vi "SistematicaAssaig.vi"(4 "Iniciar/Finalitzar":refnum<vi>, 5 "PantallaColocada":refnum<vi>, 6 "T0":refnum<vi>, 7 "Value":enum32{"Calibración", "Ensayo A", "Ensayo B"}(ring), 8 "Primera":refnum<vi>, 9 "Temperatura1":refnum<vi>, 10 "Poner Pantalla":refnum<vi>, 11 "DisparoPantalla":refnum<vi>) -> ()   [LabVIEW 2017]
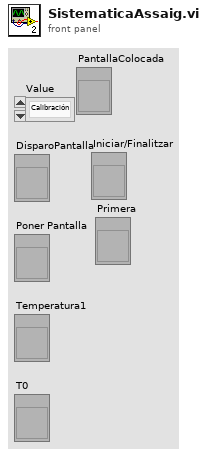
[diagram p1: front panel]
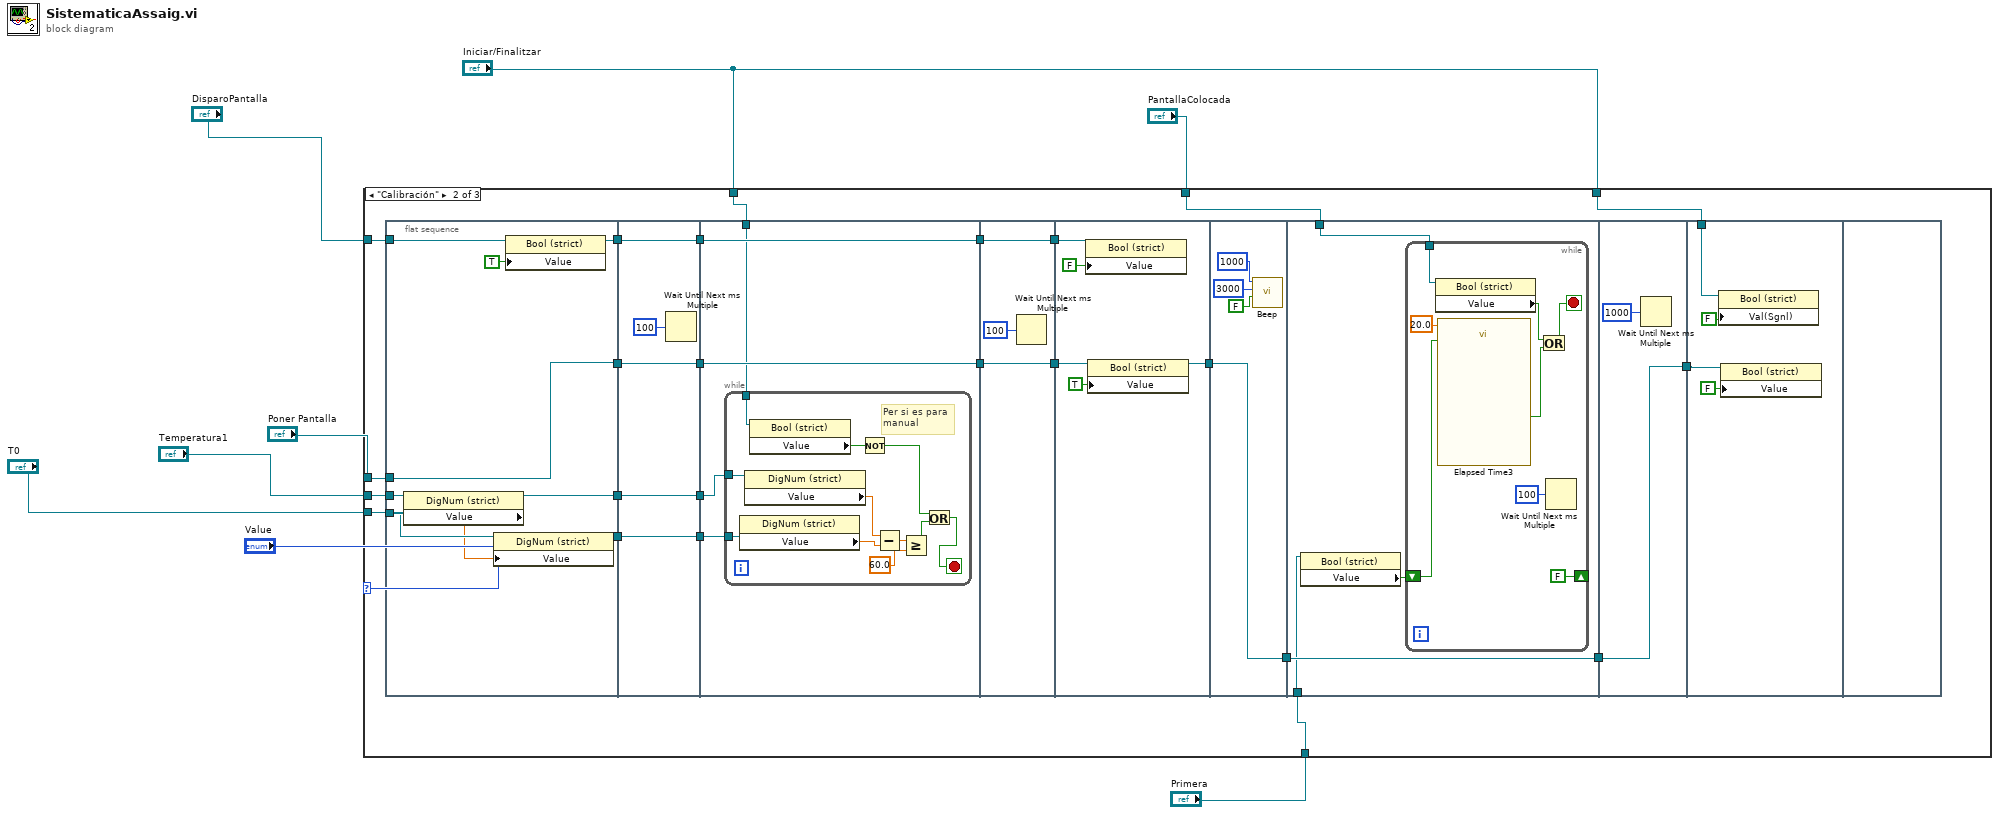
[diagram p0: block diagram]
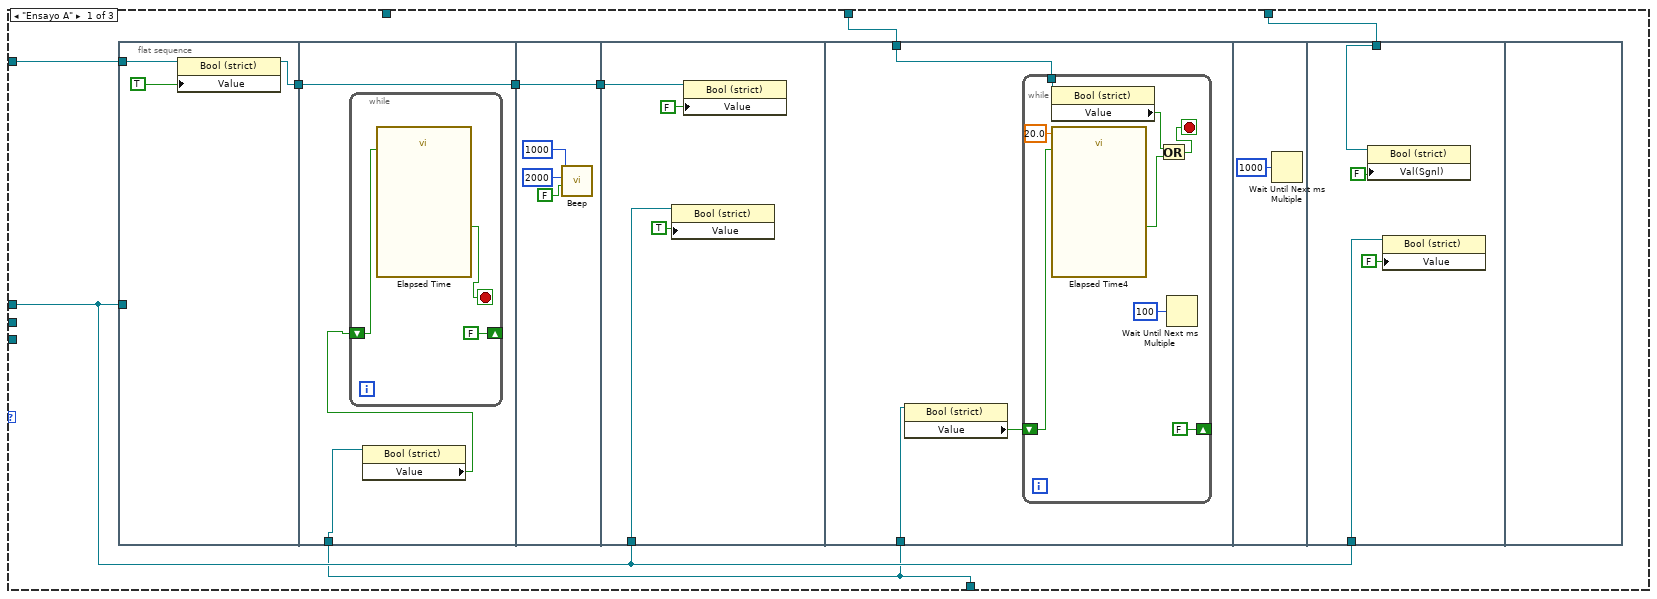
[diagram p2: hidden frame]
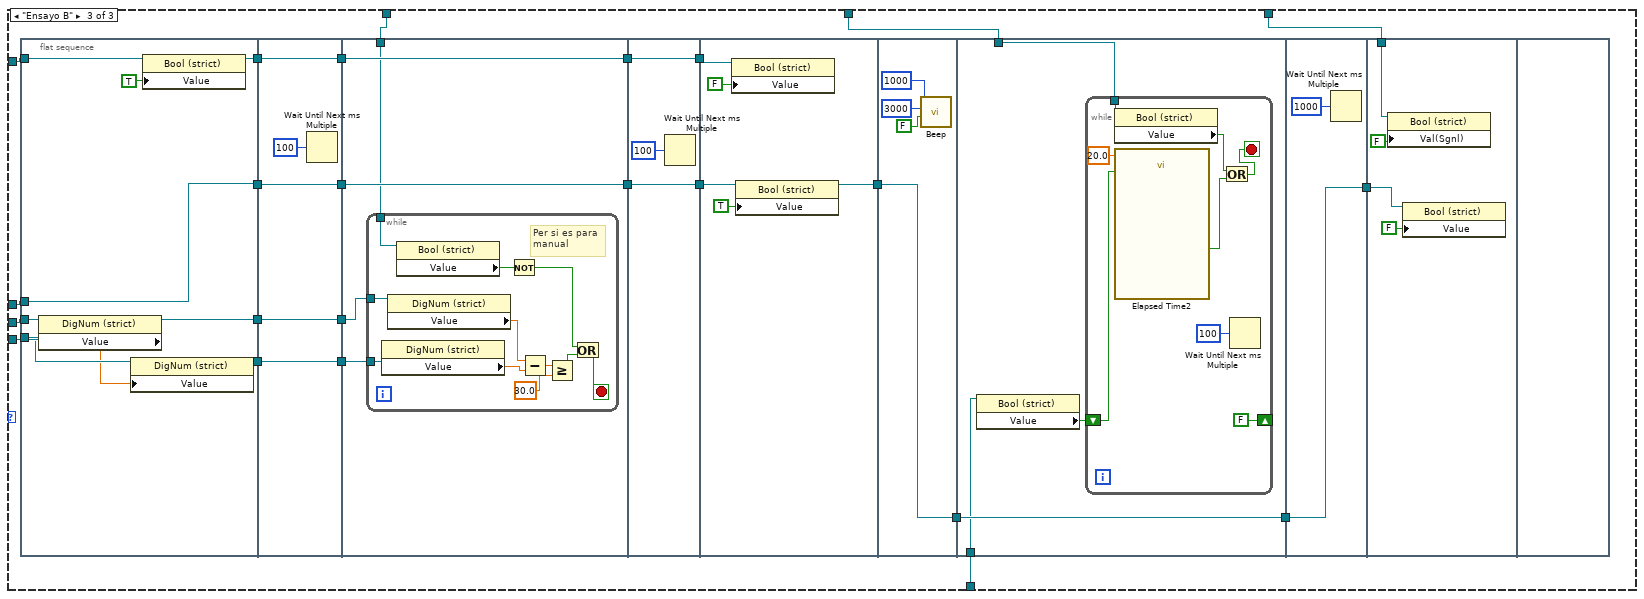
[diagram p3: hidden frame]
diagram:
  n1 = case shown="\"Calibración\"" "Value" {
    tunnel: "DisparoPantalla" -> [w16 w73 w157]
    tunnel: "Poner Pantalla" -> [w10 w71 w155]
    tunnel: "Temperatura1" -> [_ w72 w156]
    tunnel: "T0" -> [_ w70 w154]
    tunnel: "Iniciar/Finalitzar" -> [w11 w68 w152]
    tunnel: "PantallaColocada" -> [w12 w69 w153]
    tunnel: "Iniciar/Finalitzar" -> [_ w53 w137]
    tunnel: "Primera" -> [w9 w50 w134]
    frame "Ensayo A" {
      n2 = flat-sequence {
        tunnel: w16 -> [w19]
        tunnel: [w17] -> w13
        tunnel: w10 -> [_]
        tunnel: [w22] -> w14
        tunnel: w13 -> [w22]
        tunnel: w9 -> [w21]
        tunnel: [w26] -> w15
        tunnel: w14 -> [w26]
        tunnel: w15 -> [w33]
        tunnel: w10 -> [w31]
        tunnel: w12 -> [w36]
        tunnel: w9 -> [w35]
        tunnel: w11 -> [w47]
        tunnel: w10 -> [w46]
        frame #0 {
          n3 = property class="Bool (strict)"(reference=w19, "Value"=TRUE ("Reset_Time")) -> (reference out=w17:refnum<vi>)  [unwired: 1 in, 1 out]
        }
        frame #1 {
          n4 = property class="Bool (strict)"(reference=w21) -> ("Value"=w20:bool)  [unwired: 1 in, 2 out]
          n5 = while {
            shift-right: [FALSE ("Value")] -> _
            shift-left: w20 -> [w23]
            stop <- w25 stop-if-true
            n6 = call "Elapsed Time"("Reset"=w23) -> ("Time has Elapsed"=w25:bool)  [unwired: 11 in, 7 out]
          }
        }
        frame #2 {
          n7 = call <vilib>:"Beep.vi"("use system alert? (T)"=FALSE, "duration (msec)"=u32 2000, "frequency (Hz)"=u32 1000) -> ()  [unwired: 9 in]
        }
        frame #3 {
          n8 = property class="Bool (strict)"(reference=w31, "Value"=TRUE) -> ()  [unwired: 1 in, 2 out]
          n9 = property class="Bool (strict)"(reference=w33, "Value"=FALSE) -> ()  [unwired: 1 in, 2 out]
        }
        frame #4 {
          n10 = property class="Bool (strict)"(reference=w35) -> ("Value"=w34:bool)  [unwired: 1 in, 2 out]
          n11 = while {
            tunnel: w36 -> [w44]
            shift-right: [FALSE ("Value")] -> _
            shift-left: w34 -> [w37]
            stop <- w41 stop-if-true
            n12 = property class="Bool (strict)"(reference=w44) -> ("Value"=w43:bool)  [unwired: 1 in, 2 out]
            n13 = call "Elapsed Time4"("Time Target (s)"=20.0, "Reset"=w37) -> ("Time has Elapsed"=w42:bool)  [unwired: 10 in, 7 out]
            n14 = Or(x=w43, y=w42) -> (x .or. y?=w41:bool)
            n15 = Wait Until Next ms Multiple(millisecond multiple=u32 100) -> ()  [unwired: 1 out]
          }
        }
        frame #5 {
          n16 = Wait Until Next ms Multiple(millisecond multiple=u32 1000) -> ()  [unwired: 1 out]
        }
        frame #6 {
          n17 = property class="Bool (strict)"(reference=w47, "Val(Sgnl)"=FALSE ("Value (Signaling)")) -> ()  [unwired: 1 in, 2 out]
          n18 = property class="Bool (strict)"(reference=w46, "Value"=FALSE) -> ()  [unwired: 1 in, 2 out]
        }
        frame #7 {
        }
      }
    }
    frame "Calibración" {
      n19 = flat-sequence {
        tunnel: w73 -> [w82]
        tunnel: w72 -> [w81]
        tunnel: [w80] -> w67
        tunnel: w71 -> [w79]
        tunnel: [w79] -> w65
        tunnel: [w77] -> w63
        tunnel: w70 -> [w76]
        tunnel: [w74] -> w61
        tunnel: w67 -> [w87]
        tunnel: [w87] -> w66
        tunnel: w65 -> [w86]
        tunnel: [w86] -> w64
        tunnel: w63 -> [w85]
        tunnel: [w85] -> w62
        tunnel: w61 -> [w84]
        tunnel: [w84] -> w60
        tunnel: w66 -> [w92]
        tunnel: w64 -> [w91]
        tunnel: [w91] -> w59
        tunnel: w62 -> [w89]
        tunnel: w60 -> [w90]
        tunnel: [w89] -> w57
        tunnel: w53 -> [w88]
        tunnel: w59 -> [w106]
        tunnel: [w106] -> w58
        tunnel: w57 -> [w105]
        tunnel: [w105] -> w56
        tunnel: [w111] -> w52
        tunnel: w58 -> [w110]
        tunnel: w56 -> [w108]
        tunnel: w52 -> [w115]
        tunnel: [w115] -> w51
        tunnel: w69 -> [w119]
        tunnel: w51 -> [w118]
        tunnel: [w118] -> w55
        tunnel: w50 -> [w116]
        tunnel: w55 -> [w129]
        tunnel: [w129] -> w54
        tunnel: w54 -> [w132]
        tunnel: w68 -> [w131]
        frame #0 {
          n20 = property class="DigNum (strict)"(reference=w81) -> (reference out=w80:refnum<vi>, "Value"=w75:sgl)  [unwired: 1 in, 1 out]
          n21 = property class="DigNum (strict)"(reference=w76, "Value"=w75) -> (reference out=w74:refnum<vi>)  [unwired: 1 in, 1 out]
          n22 = property class="Bool (strict)"(reference=w82, "Value"=TRUE ("Reset_Time")) -> (reference out=w77:refnum<vi>)  [unwired: 1 in, 1 out]
        }
        frame #1 {
          n23 = Wait Until Next ms Multiple(millisecond multiple=u32 100) -> ()  [unwired: 1 out]
        }
        frame #2 {
          n24 = while {
            tunnel: w92 -> [w103]
            tunnel: w90 -> [w99]
            tunnel: w88 -> [w96]
            stop <- w93 stop-if-true
            # "Per si es para \nmanual"
            n25 = property class="DigNum (strict)"(reference=w99) -> ("Value"=w98:sgl)  [unwired: 1 in, 2 out]
            n26 = property class="DigNum (strict)"(reference=w103) -> ("Value"=w102:sgl)  [unwired: 1 in, 2 out]
            n27 = property class="Bool (strict)"(reference=w96) -> ("Value"=w97:bool)  [unwired: 1 in, 2 out]
            n28 = Not(x=w97) -> (.not. x?=w95:bool)
            n29 = Subtract(x=w102, y=w98) -> (x-y=w101:sgl)
            n30 = Greater Or Equal?(x=w101, y=sgl 60.0) -> (x >= y?=w94:bool)
            n31 = Or(x=w95, y=w94) -> (x .or. y?=w93:bool)
          }
        }
        frame #3 {
          n32 = Wait Until Next ms Multiple(millisecond multiple=u32 100) -> ()  [unwired: 1 out]
        }
        frame #4 {
          n33 = property class="Bool (strict)"(reference=w108, "Value"=FALSE) -> ()  [unwired: 1 in, 2 out]
          n34 = property class="Bool (strict)"(reference=w110, "Value"=TRUE) -> (reference out=w111:refnum<vi>)  [unwired: 1 in, 1 out]
        }
        frame #5 {
          n35 = call <vilib>:"Beep.vi"("use system alert? (T)"=FALSE, "duration (msec)"=u32 3000, "frequency (Hz)"=u32 1000) -> ()  [unwired: 9 in]
        }
        frame #6 {
          n36 = property class="Bool (strict)"(reference=w116) -> ("Value"=w117:bool)  [unwired: 1 in, 2 out]
          n37 = while {
            tunnel: w119 -> [w127]
            shift-right: [FALSE ("Primera")] -> _
            shift-left: w117 -> [w121]
            stop <- w124 stop-if-true
            n38 = property class="Bool (strict)"(reference=w127) -> ("Value"=w125:bool)  [unwired: 1 in, 2 out]
            n39 = call "Elapsed Time3"("Time Target (s)"=20.0, "Reset"=w121) -> ("Time has Elapsed"=w126:bool)  [unwired: 10 in, 7 out]
            n40 = Or(x=w125, y=w126) -> (x .or. y?=w124:bool)
            n41 = Wait Until Next ms Multiple(millisecond multiple=u32 100) -> ()  [unwired: 1 out]
          }
        }
        frame #7 {
          n42 = Wait Until Next ms Multiple(millisecond multiple=u32 1000) -> ()  [unwired: 1 out]
        }
        frame #8 {
          n43 = property class="Bool (strict)"(reference=w131, "Val(Sgnl)"=FALSE ("Value (Signaling)")) -> ()  [unwired: 1 in, 2 out]
          n44 = property class="Bool (strict)"(reference=w132, "Value"=FALSE) -> ()  [unwired: 1 in, 2 out]
        }
        frame #9 {
        }
      }
    }
    frame "Ensayo B" {
      n45 = flat-sequence {
        tunnel: w157 -> [w166]
        tunnel: w156 -> [w165]
        tunnel: [w164] -> w151
        tunnel: w155 -> [w163]
        tunnel: [w163] -> w149
        tunnel: [w161] -> w147
        tunnel: w154 -> [w160]
        tunnel: [w158] -> w145
        tunnel: w151 -> [w171]
        tunnel: [w171] -> w150
        tunnel: w149 -> [w170]
        tunnel: [w170] -> w148
        tunnel: w147 -> [w169]
        tunnel: [w169] -> w146
        tunnel: w145 -> [w168]
        tunnel: [w168] -> w144
        tunnel: w150 -> [w176]
        tunnel: w148 -> [w175]
        tunnel: [w175] -> w143
        tunnel: w146 -> [w173]
        tunnel: w144 -> [w174]
        tunnel: [w173] -> w141
        tunnel: w137 -> [w172]
        tunnel: w143 -> [w190]
        tunnel: [w190] -> w142
        tunnel: w141 -> [w189]
        tunnel: [w189] -> w140
        tunnel: [w195] -> w136
        tunnel: w142 -> [w194]
        tunnel: w140 -> [w192]
        tunnel: w136 -> [w199]
        tunnel: [w199] -> w135
        tunnel: w153 -> [w203]
        tunnel: w135 -> [w202]
        tunnel: [w202] -> w139
        tunnel: w134 -> [w201]
        tunnel: w139 -> [w213]
        tunnel: [w213] -> w138
        tunnel: w138 -> [w216]
        tunnel: w152 -> [w215]
        frame #0 {
          n46 = property class="DigNum (strict)"(reference=w165) -> (reference out=w164:refnum<vi>, "Value"=w159:sgl)  [unwired: 1 in, 1 out]
          n47 = property class="DigNum (strict)"(reference=w160, "Value"=w159) -> (reference out=w158:refnum<vi>)  [unwired: 1 in, 1 out]
          n48 = property class="Bool (strict)"(reference=w166, "Value"=TRUE ("Reset_Time")) -> (reference out=w161:refnum<vi>)  [unwired: 1 in, 1 out]
        }
        frame #1 {
          n49 = Wait Until Next ms Multiple(millisecond multiple=u32 100) -> ()  [unwired: 1 out]
        }
        frame #2 {
          n50 = while {
            tunnel: w176 -> [w187]
            tunnel: w174 -> [w183]
            tunnel: w172 -> [w181]
            stop <- w180 stop-if-true
            # "Per si es para \nmanual"
            n51 = property class="DigNum (strict)"(reference=w183) -> ("Value"=w182:sgl)  [unwired: 1 in, 2 out]
            n52 = property class="DigNum (strict)"(reference=w187) -> ("Value"=w186:sgl)  [unwired: 1 in, 2 out]
            n53 = property class="Bool (strict)"(reference=w181) -> ("Value"=w178:bool)  [unwired: 1 in, 2 out]
            n54 = Not(x=w178) -> (.not. x?=w177:bool)
            n55 = Subtract(x=w186, y=w182) -> (x-y=w185:sgl)
            n56 = Greater Or Equal?(x=w185, y=sgl 30.0) -> (x >= y?=w179:bool)
            n57 = Or(x=w177, y=w179) -> (x .or. y?=w180:bool)
          }
        }
        frame #3 {
          n58 = Wait Until Next ms Multiple(millisecond multiple=u32 100) -> ()  [unwired: 1 out]
        }
        frame #4 {
          n59 = property class="Bool (strict)"(reference=w192, "Value"=FALSE) -> ()  [unwired: 1 in, 2 out]
          n60 = property class="Bool (strict)"(reference=w194, "Value"=TRUE) -> (reference out=w195:refnum<vi>)  [unwired: 1 in, 1 out]
        }
        frame #5 {
          n61 = call <vilib>:"Beep.vi"("use system alert? (T)"=FALSE, "duration (msec)"=u32 3000, "frequency (Hz)"=u32 1000) -> ()  [unwired: 9 in]
        }
        frame #6 {
          n62 = property class="Bool (strict)"(reference=w201) -> ("Value"=w200:bool)  [unwired: 1 in, 2 out]
          n63 = while {
            tunnel: w203 -> [w211]
            shift-right: [FALSE ("Value")] -> _
            shift-left: w200 -> [w204]
            stop <- w208 stop-if-true
            n64 = property class="Bool (strict)"(reference=w211) -> ("Value"=w210:bool)  [unwired: 1 in, 2 out]
            n65 = call "Elapsed Time2"("Time Target (s)"=20.0, "Reset"=w204) -> ("Time has Elapsed"=w209:bool)  [unwired: 10 in, 7 out]
            n66 = Or(x=w210, y=w209) -> (x .or. y?=w208:bool)
            n67 = Wait Until Next ms Multiple(millisecond multiple=u32 100) -> ()  [unwired: 1 out]
          }
        }
        frame #7 {
          n68 = Wait Until Next ms Multiple(millisecond multiple=u32 1000) -> ()  [unwired: 1 out]
        }
        frame #8 {
          n69 = property class="Bool (strict)"(reference=w215, "Val(Sgnl)"=FALSE ("Value (Signaling)")) -> ()  [unwired: 1 in, 2 out]
          n70 = property class="Bool (strict)"(reference=w216, "Value"=FALSE) -> ()  [unwired: 1 in, 2 out]
        }
        frame #9 {
        }
      }
    }
  }
